vi "Temperature Limit.vi"() -> ()   [LabVIEW 2015]
doc: "This VI simulates the acquisition of temperature, graphs the temperature, and notifies the user if the temperature is over the limit."
panel:
  in  "Path":path
  in  "Start":bool
  in  "Delta t (ms)":i32(slide)=400 scale=50.0..500.0
  in  "Stop":bool
  in  "High Limit":dbl=28.0 format="%.2f"
  out "Temperature":cluster{"Temperature":dbl, "High Limit":dbl}(graph)={"Temperature"=85.88749999999999, "High Limit"=80.0}
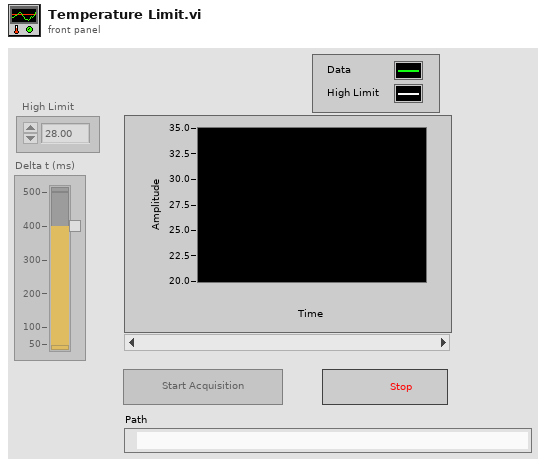
[diagram p1: front panel]
types:
  T1 = enum8{"Enabled", "Disabled", "Disabled and Grayed Out"}
  T2 = enum16{"Always On", "Always Off", "Off While Running"}
  T3 = cluster{"Temperature Value":dbl, "High Limit":dbl}
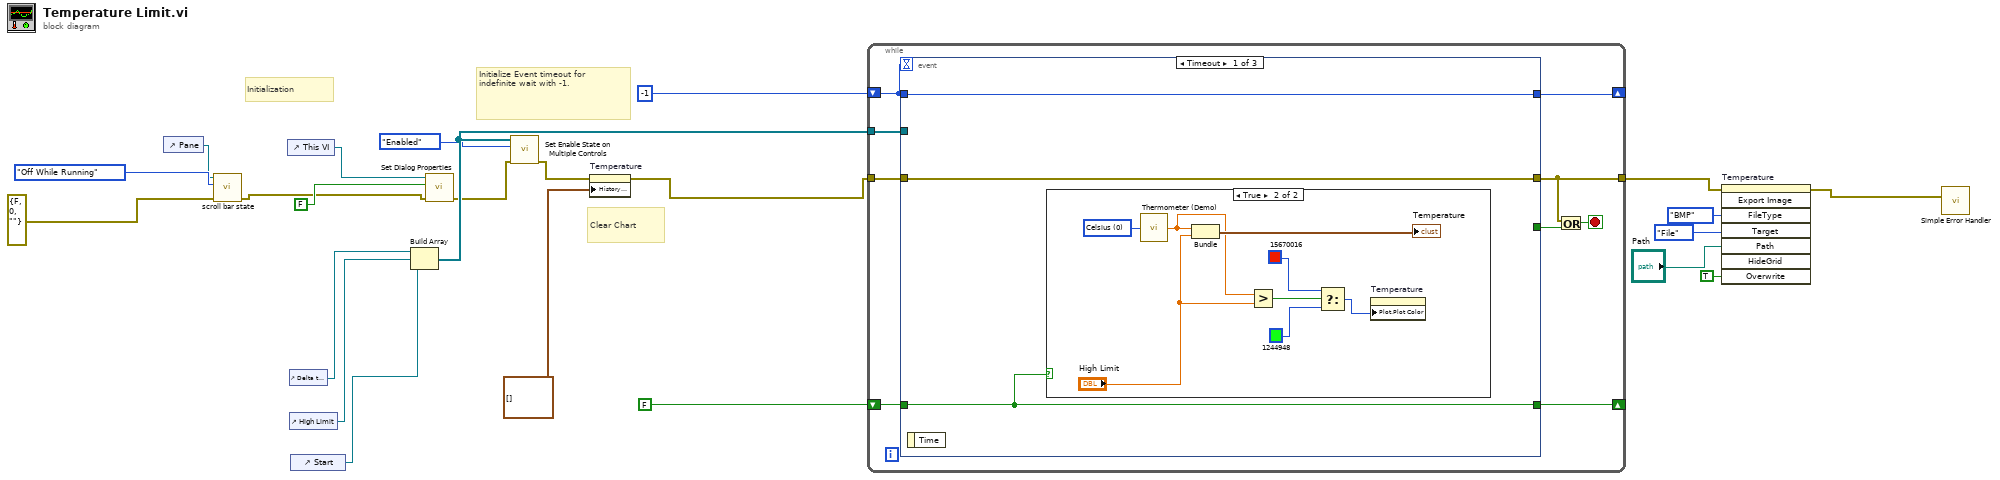
[diagram p0: block diagram]
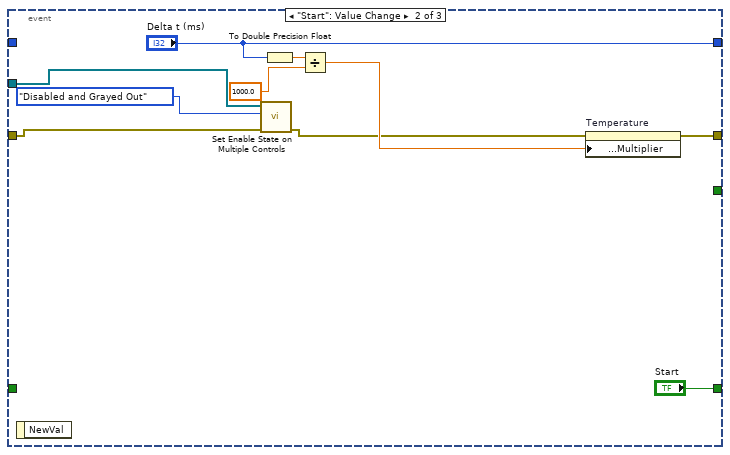
[diagram p3: hidden frame]
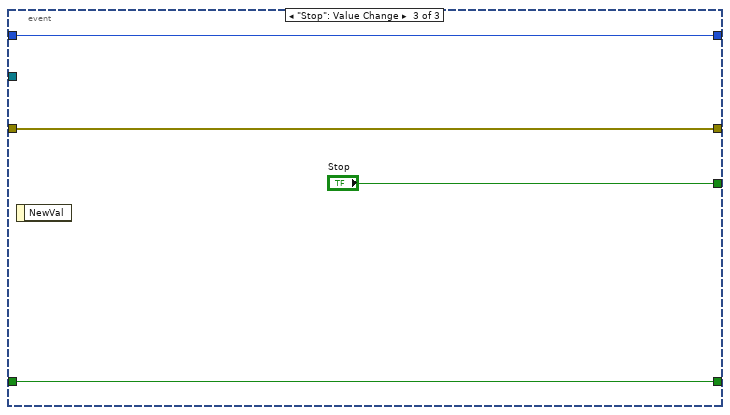
[diagram p4: hidden frame]
diagram:
  # "Clear Chart"
  # "Initialize Event timeout for indefinite wait with -1."
  # "Initialization"
  n1 = control-ref of="Pane"() -> (w15:refnum<vi>)
  n2 = call "scroll bar state.vi"("error in (no error)"=errorcluster {"status"=FALSE, "code"=0, "source"=""}, "Horizontal Scrollbar Visibility"=T2."Off While Running", "Pane ref in"=w15) -> ("error out"=w18:errorcluster)  [unwired: 8 in]
  n3 = control-ref of="This VI"() -> (w19:refnum<vi>)
  n4 = control-ref of="Delta t (ms)"() -> (w14:refnum<vi>)
  n5 = control-ref of="High Limit"() -> (w13:refnum<vi>)
  n6 = control-ref of="Start"() -> (w12:refnum<vi>)
  n7 = Build Array(w14, w13, w12) -> (w11:refnum<vi>[])
  n8 = call "Set Dialog Properties.vi"("error in (no error)"=w18, "Boolean"=FALSE, "VI in"=w19) -> ("error out"=w9:errorcluster)  [unwired: 8 in]
  n9 = call "Set Enable State on Multiple Controls.vi"("Error In"=w9, "Disabled State"=T1."Enabled", "Controls"=w11) -> ("Error Out"=w8:errorcluster)  [unwired: 8 in]
  n10 = property on="Temperature" class="WFChart (strict)"(error in=w8, "History Data"=cluster{"Temperature":dbl, "High Limit":dbl}[] []) -> (error out=w7:errorcluster)  [unwired: 1 in, 1 out]
  n11 = while {
    tunnel: w7 -> [w32]
    tunnel: [w30] -> w6
    shift-right: [w28] -> _
    shift-left: FALSE ("Start") -> [w27]
    shift-right: [w26] -> _
    shift-left: -1 ("Delta t (ms)") -> [w25]
    tunnel: w11 -> [w24]
    stop <- w31 stop-if-true
    n12 = event shown="[0] Timeout" {
      selector: _ -> [_ _ _]
      dyn-events: _ -> [_ _ _]
      timeout: w25 -> [_ _ _]
      tunnel: [_ _ "Stop"] -> w29
      tunnel: w32 -> [w35 w46 w56]
      tunnel: [w35 w53 w56] -> w30
      tunnel: [w33 "Start" w55] -> w28
      tunnel: w27 -> [w33 _ w55]
      tunnel: [w34 "Delta t (ms)" w54] -> w26
      tunnel: w25 -> [w34 _ w54]
      tunnel: w24 -> [_ w44 _]
      event Timeout {
        n13 = event-data() -> ()  [unwired: 1 in, 1 out]
        n14 = case shown="True" w33 {
          frame False {
          }
          frame True {
            w42 = u16 0 items=["Celsius", "Fahrenheit"] ("Units (0: Celsius)")
            n15 = call "Thermometer (Demo).vi"("Units (0: Celsius)"=w42) -> ("Temperature Value"=w40:dbl)
            n16 = Bundle("Temperature Value"=w40, "High Limit"="High Limit") -> (→"Temperature":T3)  [unwired: 1 in]
            n17 = Greater?(x=w40, y="High Limit") -> (0:w41:bool)
            n18 = Select(t=u32 15670016, s=w41, f=u32 1244948) -> (s? t:f=w36:u32)
            n19 = property on="Temperature" class="WFChart (strict)"("Plot.Plot Color"=w36) -> ()  [unwired: 2 in, 2 out]
          }
        }
      }
      event "Start": Value Change {
        n20 = event-data() -> ()  [unwired: 1 in, 1 out]
        n21 = call "Set Enable State on Multiple Controls.vi"("Error In"=w46, "Disabled State"=T1."Disabled and Grayed Out", "Controls"=w44) -> ("Error Out"=w45:errorcluster)  [unwired: 8 in]
        n22 = To Double Precision Float(number="Delta t (ms)") -> (double precision float=w52:dbl)
        n23 = Divide(x=w52, y=1000.0) -> (x/y=w50:dbl)
        n24 = property on="Temperature" class="WFChart (strict)"(error in=w45, "X Scale.Offset and Multiplier:Multiplier"=w50) -> (error out=w53:errorcluster)  [unwired: 1 in, 1 out]
      }
      event "Stop": Value Change {
        n25 = event-data() -> ()  [unwired: 1 in, 1 out]
      }
    }
    n26 = Or(x=w30, y=w29) -> (x .or. y?=w31:bool)
  }
  n27 = invoke on="Temperature" class="WFChart (strict)" method="Export Image"(error in=w6, "FileType"=enum32{"BMP", "EPS", "EMF", "PICT"}."BMP" ("File Type"), "Target"=enum32{"File", "Clipboard"}."File", "Path"="Path", "Overwrite"=TRUE ("Always Overwrite")) -> (error out=w5:errorcluster)  [unwired: 3 in, 7 out]
  n28 = call <vilib>:"Simple Error Handler.vi"("error in (no error)"=w5) -> ()  [unwired: 4 in, 5 out]
